vi "FTW-Test-JSON-AtomicIncrement.vi"() -> (0 "Test Result":errorcluster)   [LabVIEW 2015]
uses:
  src/json/FTW-JSON-Type.ctl
  src/json/core/FTW-JSON-Core-Type.ctl
  lib/FTW-KernelFilepath.vi
  src/json/core/FTW-JSON-Core-LibraryReturnValue.vi
  src/error/FTW-ERR-ThrowInvalidReferenceError.vi
  src/json/core/FTW-JSON-Core-ElementType.vi
  codegen/xnode/FTW-JSON-Fetch.xnode
  src/core/type/FTW-Type-JSON.ctl
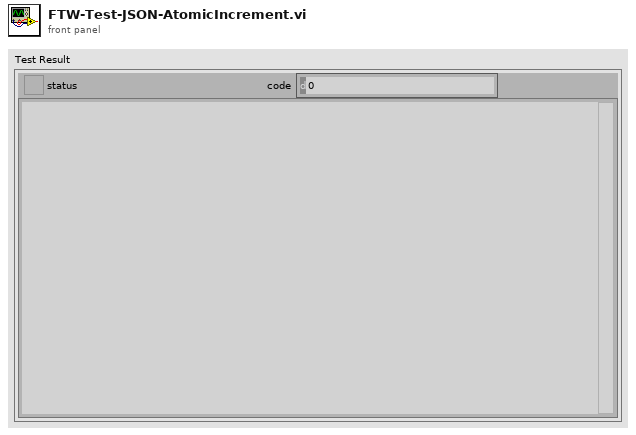
[diagram p1: front panel]
types:
  T1 = typedef "FTW-JSON-Type.ctl" = enum8{"Not Found", "Object", "Array", "String", "Number", "Boolean", "null"}
  T2 = typedef "FTW-Type-JSON.ctl" = refnum<data-value>
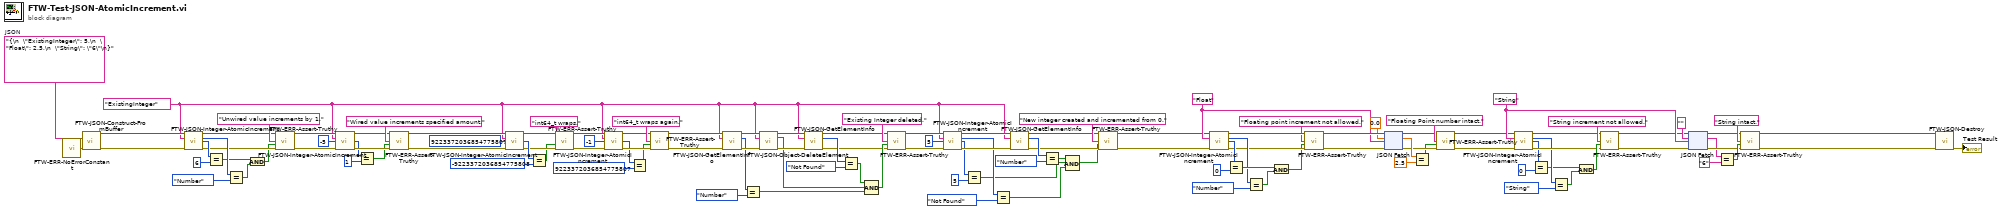
[diagram p0: block diagram]
diagram:
  w52 = "String" ("Path to Integer")
  w65 = "Float" ("Path to Integer")
  w15 = "ExistingInteger" ("Path to Integer")
  w112 = "{\n  \"ExistingInteger\": 5,\n  \"Float\": 2.5,\n  \"String\": \"6\"\n}"  # JSON
  n1 = call "FTW-ERR-NoErrorConstant.vi"() -> ("no error"=w114:errorcluster)
  n2 = call "FTW-JSON-Construct-FromBuffer.vi"("JSON String (UTF-8)"=w112, "error in"=w114) -> ("JSON"=w111:T2, "error out"=w110:errorcluster)  [unwired: 12 in]
  n3 = call "FTW-JSON-Integer-AtomicIncrement.vi"("JSON"=w111, "Path to Integer"=w15, "error in"=w110) -> ("JSON out"=w101:T2, "Original Element Type"=w109:T1, "New Value"=w107:i64, "error out"=w103:errorcluster)  [unwired: 9 in]
  n4 = Equal?(x=w107, y=i64 6) -> (x = y?=w105:bool)
  n5 = Equal?(x=w109, y=FTW-JSON-Type."Number" ("Original Element Type")) -> (x = y?=w104:bool)
  n6 = And(x=w105, y=w104) -> (x .and. y?=w99:bool)
  n7 = call "FTW-ERR-Assert-Truthy.vi"("Assertion"="Unwired value increments by 1.", "Assertion holds true?"=w99, "error in"=w103) -> ("error out"=w100:errorcluster)  [unwired: 12 in]
  n8 = call "FTW-JSON-Integer-AtomicIncrement.vi"("JSON"=w101, "Path to Integer"=w15, "Increment"=i64 -5, "error in"=w100) -> ("JSON out"=w92:T2, "New Value"=w96:i64, "error out"=w97:errorcluster)  [unwired: 8 in, 1 out]
  n9 = Equal?(x=w96, y=i64 1) -> (x = y?=w94:bool)
  n10 = call "FTW-ERR-Assert-Truthy.vi"("Assertion"="Wired value increments specified amount.", "Assertion holds true?"=w94, "error in"=w97) -> ("error out"=w90:errorcluster)  [unwired: 12 in]
  n11 = call "FTW-JSON-Integer-AtomicIncrement.vi"("JSON"=w92, "Path to Integer"=w15, "Increment"=i64 9223372036854775807, "error in"=w90) -> ("JSON out"=w84:T2, "New Value"=w89:i64, "error out"=w87:errorcluster)  [unwired: 8 in, 1 out]
  n12 = Equal?(x=w89, y=i64 -9223372036854775808 ("Increment")) -> (x = y?=w85:bool)
  n13 = call "FTW-ERR-Assert-Truthy.vi"("Assertion"="int64_t wraps.", "Assertion holds true?"=w85, "error in"=w87) -> ("error out"=w83:errorcluster)  [unwired: 12 in]
  n14 = call "FTW-JSON-Integer-AtomicIncrement.vi"("JSON"=w84, "Path to Integer"=w15, "Increment"=i64 -1, "error in"=w83) -> ("JSON out"=w31:T2, "New Value"=w78:i64, "error out"=w79:errorcluster)  [unwired: 8 in, 1 out]
  n15 = Equal?(x=w78, y=i64 9223372036854775807 ("Increment")) -> (x = y?=w77:bool)
  n16 = call "FTW-ERR-Assert-Truthy.vi"("Assertion"="int64_t wraps again.", "Assertion holds true?"=w77, "error in"=w79) -> ("error out"=w29:errorcluster)  [unwired: 12 in]
  n17 = call "FTW-JSON-GetElementInfo.vi"("JSON"=w31, "Path to Element"=w15, "error in"=w29) -> ("JSON out"=w30:T2, "Element Type"=w26:T1, "error out"=w28:errorcluster)  [unwired: 9 in, 1 out]
  n18 = Equal?(x=w26, y=FTW-JSON-Type."Number") -> (x = y?=w24:bool)
  n19 = call "FTW-JSON-Object-DeleteElement.vi"("JSON"=w30, "Key"=w15, "error in"=w28) -> ("JSON out"=w35:T2, "Found and Removed?"=w25:bool, "error out"=w32:errorcluster)  [unwired: 10 in]
  n20 = call "FTW-JSON-GetElementInfo.vi"("JSON"=w35, "Path to Element"=w15, "error in"=w32) -> ("JSON out"=w20:T2, "Element Type"=w34:T1, "error out"=w21:errorcluster)  [unwired: 9 in, 1 out]
  n21 = Equal?(x=w34, y=FTW-JSON-Type."Not Found") -> (x = y?=w23:bool)
  n22 = Compound Arithmetic op=AND(w23, w25, w24) -> (w22:bool)
  n23 = call "FTW-ERR-Assert-Truthy.vi"("Assertion"="Existing Integer deleted.", "Assertion holds true?"=w22, "error in"=w21) -> ("error out"=w19:errorcluster)  [unwired: 12 in]
  n24 = call "FTW-JSON-Integer-AtomicIncrement.vi"("JSON"=w20, "Path to Integer"=w15, "Increment"=i64 5, "error in"=w19) -> ("JSON out"=w17:T2, "Original Element Type"=w13:T1, "New Value"=w12:i64, "error out"=w16:errorcluster)  [unwired: 8 in]
  n25 = Equal?(x=w12, y=i64 5) -> (x = y?=w3:bool)
  n26 = Equal?(x=w13, y=FTW-JSON-Type."Not Found") -> (x = y?=w2:bool)
  n27 = call "FTW-JSON-GetElementInfo.vi"("JSON"=w17, "Path to Element"=w15, "error in"=w16) -> ("JSON out"=w6:T2, "Element Type"=w10:T1, "error out"=w7:errorcluster)  [unwired: 9 in, 1 out]
  n28 = Equal?(x=w10, y=FTW-JSON-Type."Number") -> (x = y?=w4:bool)
  n29 = Compound Arithmetic op=AND(w4, w3, w2) -> (w1:bool)
  n30 = call "FTW-ERR-Assert-Truthy.vi"("Assertion"="New integer created and incremented from 0.", "Assertion holds true?"=w1, "error in"=w7) -> ("error out"=w5:errorcluster)  [unwired: 12 in]
  n31 = call "FTW-JSON-Integer-AtomicIncrement.vi"("JSON"=w6, "Path to Integer"=w65, "error in"=w5) -> ("JSON out"=w70:T2, "Original Element Type"=w71:T1, "New Value"=w72:i64, "error out"=w69:errorcluster)  [unwired: 9 in]
  n32 = Equal?(x=w72, y=i64 0) -> (x = y?=w74:bool)
  n33 = Equal?(x=w71, y=FTW-JSON-Type."Number" ("Original Element Type")) -> (x = y?=w73:bool)
  n34 = And(x=w74, y=w73) -> (x .and. y?=w66:bool)
  n35 = call "FTW-ERR-Assert-Truthy.vi"("Assertion"="Floating point increment not allowed.", "Assertion holds true?"=w66, "error in"=w69) -> ("error out"=w68:errorcluster)  [unwired: 12 in]
  n36 = xnode "JSON Fetch"("JSON"=w70, "Element Type and Default Value"=0.0 ("y"), "Element Path"=w65, "error in"=w68) -> ("JSON out"=w38:T2, "Value"=w62:dbl, "error out"=w61:errorcluster)  [unwired: 1 in, 1 out]
  n37 = Equal?(x=w62, y=2.5) -> (x = y?=w59:bool)
  n38 = call "FTW-ERR-Assert-Truthy.vi"("Assertion"="Floating Point number intact.", "Assertion holds true?"=w59, "error in"=w61) -> ("error out"=w40:errorcluster)  [unwired: 12 in]
  n39 = call "FTW-JSON-Integer-AtomicIncrement.vi"("JSON"=w38, "Path to Integer"=w52, "error in"=w40) -> ("JSON out"=w47:T2, "Original Element Type"=w46:T1, "New Value"=w45:i64, "error out"=w48:errorcluster)  [unwired: 9 in]
  n40 = Equal?(x=w45, y=i64 0) -> (x = y?=w43:bool)
  n41 = Equal?(x=w46, y=FTW-JSON-Type."String" ("Original Element Type")) -> (x = y?=w44:bool)
  n42 = And(x=w43, y=w44) -> (x .and. y?=w51:bool)
  n43 = call "FTW-ERR-Assert-Truthy.vi"("Assertion"="String increment not allowed.", "Assertion holds true?"=w51, "error in"=w48) -> ("error out"=w49:errorcluster)  [unwired: 12 in]
  n44 = xnode "JSON Fetch"("JSON"=w47, "Element Type and Default Value"="" ("y"), "Element Path"=w52, "error in"=w49) -> ("JSON out"=w37:T2, "Value"=w55:string, "error out"=w56:errorcluster)  [unwired: 1 in, 1 out]
  n45 = Equal?(x=w55, y="6") -> (x = y?=w58:bool)
  n46 = call "FTW-ERR-Assert-Truthy.vi"("Assertion"="String intact.", "Assertion holds true?"=w58, "error in"=w56) -> ("error out"=w39:errorcluster)  [unwired: 12 in]
  n47 = call "FTW-JSON-Destroy.vi"("JSON"=w37, "error in"=w39) -> ("error out"=→"Test Result":errorcluster)  [unwired: 13 in]
